vi "Find Distances.vi"(7 "Maze":refnum<class "Maze.lvclass">, 11 "Mouse in":refnum<class "Mouse.lvclass">) -> (3 "Mouse out":refnum<class "Mouse.lvclass">)   [LabVIEW 2020, in "Maze.lvlib" / "Mouse.lvclass"]
uses:
  Mouse.lvclass
  Maze/Maze.lvclass
  Distances.ctl
  Mouse.lvclass/Mouse.ctl
  Maze.lvlib
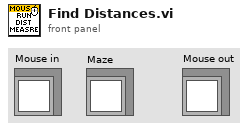
[diagram p1: front panel]
types:
  T1 = typedef "Maze.lvlib/Distances.ctl" = cluster{"Forward":i32, "Back":i32, "Left":i32, "Right":i32}
  T2 = typedef "Maze.lvlib/Position.ctl" = cluster{"S":i32, "E":i32}
  T3 = typedef "Maze.lvlib/Direction.ctl" = enum8{"East", "North", "West", "South"}
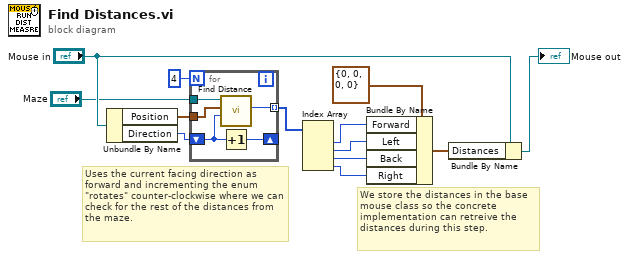
[diagram p0: block diagram]
diagram:
  # "We store the distances in the base mouse class so the concrete implementation can retreive the distances during this step."
  # "Uses the current facing direction as forward and incrementing the enum \"rotates\" counter-clockwise where we can check for the rest of the distances from the maze."
  n1 = Unbundle By Name("Mouse in") -> ("Position"=w12:T2, "Direction"=w10:T3)
  n2 = for {
    N: 4 -> [_]
    tunnel: "Maze" -> [w18]
    tunnel: w12 -> [w16]
    shift-right: [w17] -> _
    shift-left: w10 -> [w15]
    tunnel: [w14] -> w8 mode=indexing
    n3 = call "Find Distance.vi"("Direction"=w15, "Position"=w16, "Maze in"=w18) -> ("Distance"=w14:i32)  [unwired: 7 in, 1 out]
    n4 = Increment(x=w15) -> (x+1=w17:T3)
  }
  n5 = Index Array(array=w8) -> (element #1=w7:i32, element #2=w5:i32, element #3=w6:i32, element #4=w4:i32)  [unwired: 4 in]
  n6 = Bundle By Name(cluster=T1 {"Forward"=0, "Back"=0, "Left"=0, "Right"=0} ("Distances"), "Forward"=w7, "Left"=w5, "Back"=w6, "Right"=w4) -> (w2:T1)
  n7 = Bundle By Name(cluster="Mouse in", "Distances"=w2) -> (→"Mouse out":refnum<class "Mouse.lvclass">)
